vi "Format Child Table of Contents.vi"(4 "Include":string[](array[string]), 6 "Exclude":string[](array[string]), 7 "Printable?":bool caption="All? (T)", 8 "Error in":errorcluster caption="Error in (no error)", 9 "Min Level":i32=1, 10 "Depth":i32=6, 11 "Style":T1 caption="Style (Default)") -> (0 "Error out":errorcluster, 3 "Table of Contents String":string)   [LabVIEW 2023, in "Confluence Formatting.lvlib"]
uses:
  Confluence Formatting.lvlib
  Types/Table of Contents Style.ctl
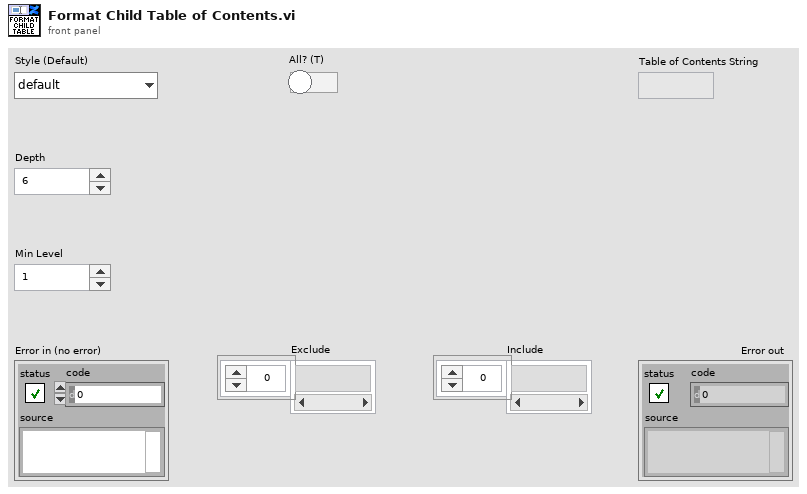
[diagram p1: front panel]
types:
  T1 = typedef "Confluence Formatting.lvlib/Table of Contents Style.ctl" = enum16{"default", "disc", "square", "none"}
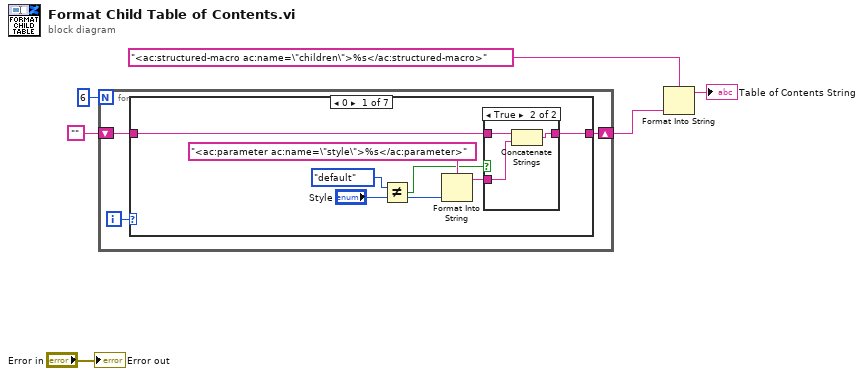
[diagram p0: block diagram]
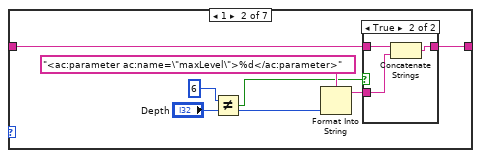
[diagram p3: hidden frame]
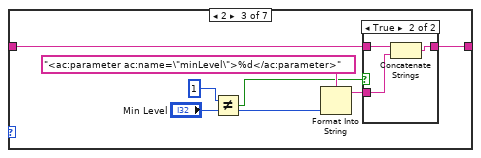
[diagram p5: hidden frame]
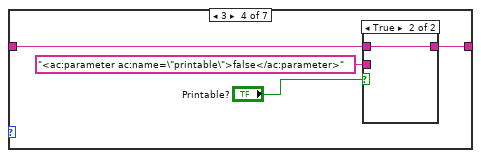
[diagram p7: hidden frame]
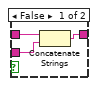
[diagram p8: hidden frame]
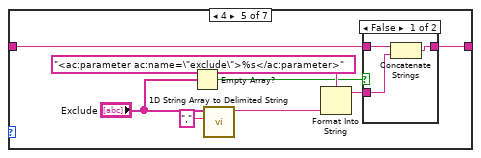
[diagram p9: hidden frame]
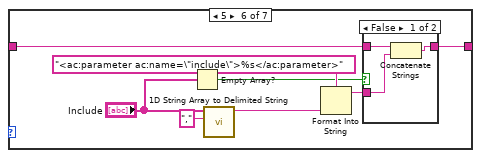
[diagram p11: hidden frame]
diagram:
  n1 = for {
    N: 6 -> [_]
    shift-right: [w7] -> w1
    shift-left: "" -> [w8]
    i -> [w9]
    n2 = case shown="0" w9 {
      tunnel: w8 -> [w13 w25 w36 w45 w56 w68 w75]
      tunnel: [w14 w26 w37 w46 w57 w69 w75] -> w7
      frame 0 {
        n3 = Not Equal?(x=Table_of_Contents_Style."default" ("y"), y="Style") -> (x != y?=w10:bool)
        n4 = Format Into String(format string="<ac:parameter ac:name=\"style\">%s</ac:parameter>", "Style") -> (resulting string=w11:string)  [unwired: 2 in, 1 out]
        n5 = case shown="True" w10 {
          tunnel: [w17 w20] -> w14
          tunnel: w13 -> [w17 w19]
          tunnel: w11 -> [_ w18]
          frame False {
          }
          frame True {
            n6 = Concatenate Strings(w19, w18) -> (w20:string)
          }
        }
      }
      frame 1 {
        n7 = Not Equal?(x=6, y="Depth") -> (x != y?=w23:bool)
        n8 = Format Into String(format string="<ac:parameter ac:name=\"maxLevel\">%d</ac:parameter>", "Depth") -> (resulting string=w24:string)  [unwired: 2 in, 1 out]
        n9 = case shown="True" w23 {
          tunnel: [w28 w31] -> w26
          tunnel: w25 -> [w28 w30]
          tunnel: w24 -> [_ w29]
          frame False {
          }
          frame True {
            n10 = Concatenate Strings(w30, w29) -> (w31:string)
          }
        }
      }
      frame 2 {
        n11 = Not Equal?(x=1, y="Min Level") -> (x != y?=w34:bool)
        n12 = Format Into String(format string="<ac:parameter ac:name=\"minLevel\">%d</ac:parameter>", "Min Level") -> (resulting string=w35:string)  [unwired: 2 in, 1 out]
        n13 = case shown="True" w34 {
          tunnel: [w39 w42] -> w37
          tunnel: w36 -> [w39 w41]
          tunnel: w35 -> [_ w40]
          frame False {
          }
          frame True {
            n14 = Concatenate Strings(w41, w40) -> (w42:string)
          }
        }
      }
      frame 3 {
        n15 = case shown="True" "Printable?" {
          tunnel: [w49 w50] -> w46
          tunnel: w45 -> [w48 w50]
          tunnel: "<ac:parameter ac:name=\"printable\">false</ac:parameter>" ("format string") -> [w47 _]
          frame False {
            n16 = Concatenate Strings(w48, w47) -> (w49:string)
          }
          frame True {
          }
        }
      }
      frame 4 {
        n17 = Empty Array?(array="Exclude") -> (empty?=w54:bool)
        n18 = call <vilib>:"1D String Array to Delimited String.vi"("delimiter"=",", "string array"="Exclude") -> ("delimited string"=w52:string)  [unwired: 9 in]
        n19 = Format Into String(format string="<ac:parameter ac:name=\"exclude\">%s</ac:parameter>", w52) -> (resulting string=w55:string)  [unwired: 2 in, 1 out]
        n20 = case shown="False" w54 {
          tunnel: [w61 w62] -> w57
          tunnel: w56 -> [w60 w62]
          tunnel: w55 -> [w59 _]
          frame False {
            n21 = Concatenate Strings(w60, w59) -> (w61:string)
          }
          frame True {
          }
        }
      }
      frame 5 {
        n22 = Empty Array?(array="Include") -> (empty?=w66:bool)
        n23 = call <vilib>:"1D String Array to Delimited String.vi"("delimiter"=",", "string array"="Include") -> ("delimited string"=w65:string)  [unwired: 9 in]
        n24 = Format Into String(format string="<ac:parameter ac:name=\"include\">%s</ac:parameter>", w65) -> (resulting string=w67:string)  [unwired: 2 in, 1 out]
        n25 = case shown="False" w66 {
          tunnel: [w73 w74] -> w69
          tunnel: w68 -> [w72 w74]
          tunnel: w67 -> [w71 _]
          frame False {
            n26 = Concatenate Strings(w72, w71) -> (w73:string)
          }
          frame True {
          }
        }
      }
      frame Default {
      }
    }
  }
  n27 = Format Into String(format string="<ac:structured-macro ac:name=\"children\">%s</ac:structured-macro>", w1) -> (resulting string=→"Table of Contents String":string)  [unwired: 2 in, 1 out]
  "Error out" <- "Error in"
